vi "test - Get Filter String - 1.vi"(8 "error in (no error)":errorcluster, 11 "TestCase in":refnum<class "Time Filter Tester.lvclass">) -> (0 "error out":errorcluster, 3 "TestCase out":refnum<class "Time Filter Tester.lvclass">)   [LabVIEW 2016, in "Assert API Components.lvlib" / "Time Filter Tester.lvclass"]
uses:
  Time Filter Tester.lvclass
  Time Filter Tester.lvclass/Time Filter Tester.ctl
  Core/Assert API Components/Filter Configurations/Time Filters/Time Filters.lvclass
  <vilib>/addons/_JKI Toolkits/VI Tester/TestCase.llb/TestCase.lvclass
  C:/Program Files (x86)/National Instruments/LabVIEW 2016/vi.lib/addons/_JKI Toolkits/VI Tester/TestCase.llb/TestCase.lvclass
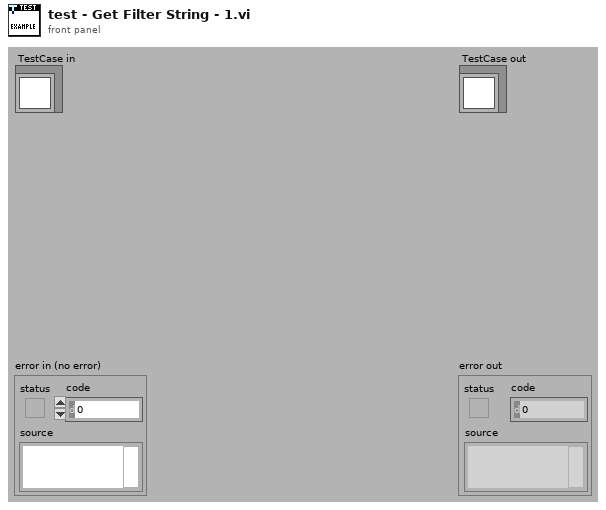
[diagram p1: front panel]
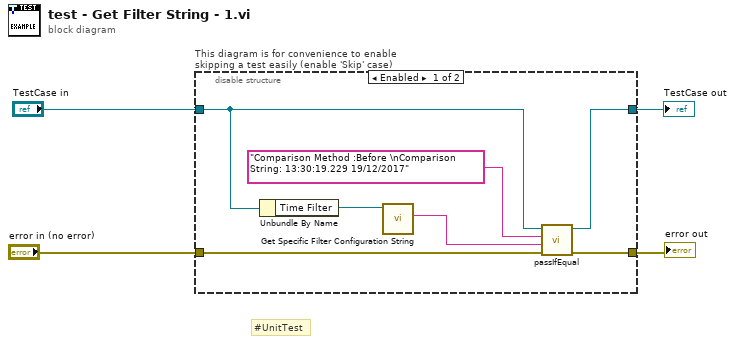
[diagram p0: block diagram]
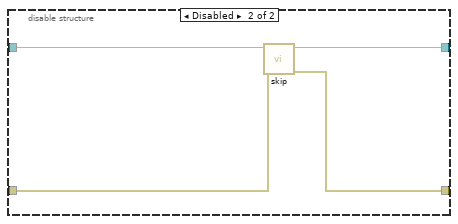
[diagram p2: hidden frame]
diagram:
  # "#UnitTest"
  n1 = disable-structure "This diagram is for convenience to enable skipping a test easily (enable 'Skip' case)" shown="Enabled" {
    disable-tunnel: "TestCase in" -> [w9 w15]
    disable-tunnel: [w11 w13] -> w1
    disable-tunnel: [w10 w14] -> w3
    disable-tunnel: "error in (no error)" -> [w6 w12]
    frame Enabled {
      n2 = Unbundle By Name(w9) -> ("Time Filter"=w8:refnum<class "Time Filters.lvclass">)
      n3 = call-dynamic "Get Specific Filter Configuration String.vi"("Time Filters in"=w8) -> ("Filter String"=w7:string)  [unwired: 10 in]
      n4 = call-dynamic "passIfEqual.vi"("error in (no error)"=w6, "y"=w7, "x"="Comparison Method :Before \nComparison String: 13:30:19.229 19/12/2017", "TestCase in"=w9) -> ("error out"=w10:errorcluster, "TestCase out"=w11:refnum<class "Time Filter Tester.lvclass">)  [unwired: 6 in]
    }
    frame Disabled {
      # "skip test result while test is under development"
      n5 = call <vilib>:"skip.vi"("error in (no error)"=w12, "TestCase in"=w15) -> ("error out"=w14:errorcluster, "TestCase out"=w13:refnum<class "Time Filter Tester.lvclass">)  [unwired: 8 in]
    }
  }
  "error out" <- w3
  "TestCase out" <- w1
